vi "Write Data to Log File Instance (U8).vi"(6 "Data":u8[][](array[numeric]), 8 "error in (no error)":errorcluster, 9 "Channel Names":string[](array[string]), 10 "Group Names":string[](array[string]), 11 "Segmented Log in":refnum<class "Segmented Log.lvclass">) -> (0 "error out":errorcluster, 2 "Log Active":bool, 3 "Segmented Log out":refnum<class "Segmented Log.lvclass">)   [LabVIEW 2015, in "Waveform Data Logger Engine.lvlib" / "Segmented Log.lvclass"]
doc: "Writes data to a log file instance. If the segmented log is still active, ensures a valid file instance is open before logging data. After each write operation, checks if the current file instance has surpassed any limits and needs to be closed."
uses:
  Segmented Log.lvclass
  Segmented Log.lvclass/Segmented Log.ctl
  Shared/Classes/Log File Specifications/Log File Specification/Log File Specification.lvclass/Log File Specification.ctl
  Footprint Segmented Log/Footprint Segmented Log.lvclass/Footprint Segmented Log.ctl
  Log Files/Log File/Log File.lvclass/Log File.ctl
  Time Segmented Log/Time Segmented Log.lvclass/Time Segmented Log.ctl
  Log Files/TDMS Log File/TDMS Log File.lvclass/TDMS Log File.ctl
  Log Files/Text Log File/Text Log File.lvclass/Text Log File.ctl
  Close Log File Instance.vi
  Segment Log File.vi
  Open Log File Instance.vi
  Log Files/Log File/Close Log File.vi
  Make File Read-Only.vi
  On Segmented Log Complete.vi
  On File Close.vi
  Footprint Segmented Log/Segment Log File (Footprint).vi
  Time Segmented Log/Segment Log File (Time).vi
  Shared/Classes/Log File Specifications/Log File Specification/Open Log File.vi
  Shared/Classes/Log File Specifications/Log File Specification/Set Path Tag.vi
  On File Open.vi
  Shared/Classes/Log File Specifications/Log File Specification/Set Filename Offset.vi
  Log Files/TDMS Log File/Close TDMS Log File.vi
  Log Files/Text Log File/Close Text Log File.vi
  Get Current Log File Instance.vi
  Log Files/Log File/Get File Size.vi
  Log Files/Log File/Get Start Time.vi
  Shared/Classes/Log File Specifications/Log File Specification/Build File Path.vi
  Shared/Classes/Log File Specifications/Log File Specification/Resolve File Conflicts.vi
  <vilib>/Utility/error.llb/Error Cluster From Error Code.vi
  Shared/Classes/Log File Specifications/Log File Specification/Initialize Log File.vi
  <vilib>/Utility/libraryn.llb/Create Directory Recursive.vi
  <vilib>/Utility/libraryn.llb/Check if File or Folder Exists.vi
  <vilib>/Utility/libraryn.llb/Get File Extension.vi
  Log Files/Text Log File/Text Log File.lvclass
  Log Files/TDMS Log File/TDMS Log File.lvclass
  Log Files/Log File/Log File.lvclass
  Time Segmented Log/Time Segmented Log.lvclass
  Footprint Segmented Log/Footprint Segmented Log.lvclass
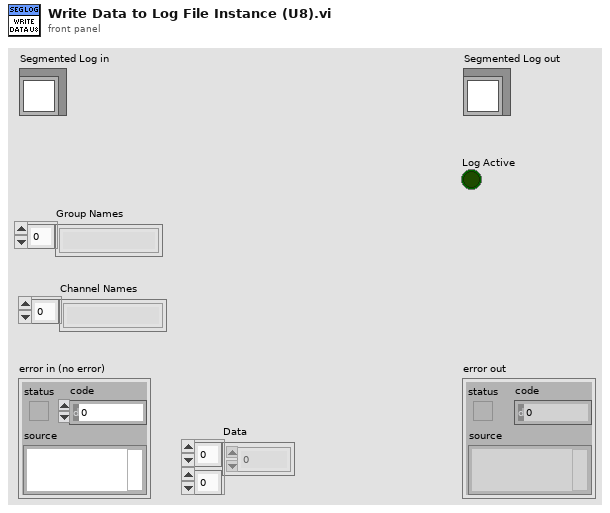
[diagram p1: front panel]
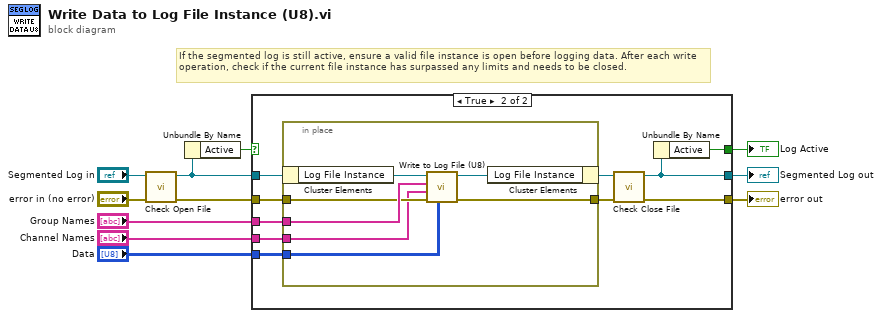
[diagram p0: block diagram]
diagram:
  # "If the segmented log is still active, ensure a valid file instance is open before logging data. After each write operation, check if the current file instance has surpassed any limits and needs to be closed."
  n1 = call "Check Open File.vi"("error in (no error)"="error in (no error)", "Segmented Log in"="Segmented Log in") -> ("error out"=w3:errorcluster, "Segmented Log out"=w2:refnum<class "Segmented Log.lvclass">)  [unwired: 8 in]
  n2 = Unbundle By Name(w2) -> ("Active"=w1:bool)
  n3 = case shown="True" w1 {
    selector: w1 -> [w12 _]
    tunnel: "Group Names" -> [_ w24]
    tunnel: w3 -> [w13 w20]
    tunnel: "Channel Names" -> [_ w19]
    tunnel: "Data" -> [_ w23]
    tunnel: [w14 w16] -> w8
    tunnel: [w13 w21] -> w10
    tunnel: w2 -> [w14 w18]
    tunnel: [w12 w15] -> w4
    frame False {
      # "This segmented logging configuration is no longer active."
    }
    frame True {
      n4 = in-place {
        in-place-border: w24 -> [w31]
        in-place-border: w23 -> [w30]
        in-place-border: [w29] -> w22
        in-place-border: w20 -> [w28]
        in-place-border: w19 -> [w27]
        n5 = in-place-cluster #1(w18) -> ("Log File Instance"=w26:refnum<class "Log File.lvclass">)
        n6 = call "Write to Log File (U8).vi"("Data"=w30, "error in (no error)"=w28, "Channel Names in"=w27, "Group Names in"=w31, "Log File in"=w26) -> ("error out"=w29:errorcluster, "Log File out"=w25:refnum<class "Log File.lvclass">)  [unwired: 5 in]
        n7 = in-place-cluster #1("Log File Instance"=w25) -> (w17:refnum<class "Segmented Log.lvclass">)
      }
      n8 = call "Check Close File.vi"("error in (no error)"=w22, "Segmented Log in"=w17) -> ("error out"=w21:errorcluster, "Segmented Log out"=w16:refnum<class "Segmented Log.lvclass">)  [unwired: 8 in]
      n9 = Unbundle By Name(w16) -> ("Active"=w15:bool)
    }
  }
  "error out" <- w10
  "Segmented Log out" <- w8
  "Log Active" <- w4
